vi "CreateShift.vi"(7 "Shifter Name":string, 8 "error in (no error)":errorcluster, 9 "Duration Hours":u8, 10 "Start Hour":u8, 11 "Date":string) -> (0 "error out":errorcluster, 3 "Shift":refnum<class "Shift.lvclass">)   [LabVIEW 2013, in "Shift Schedule.lvclass"]
uses:
  Shift Schedule.lvclass
  Shift.lvclass
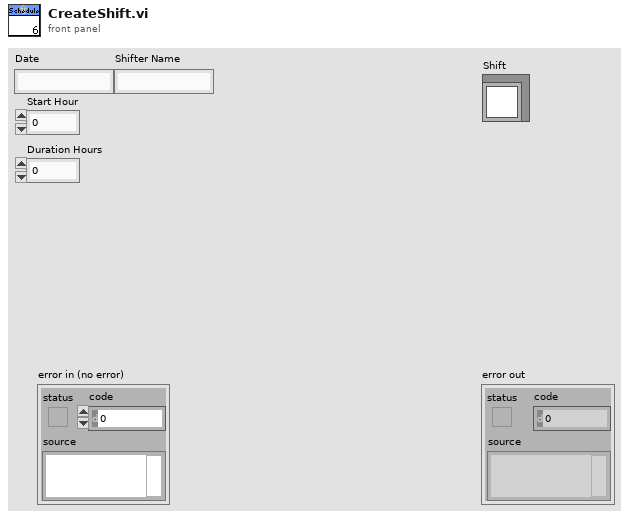
[diagram p1: front panel]
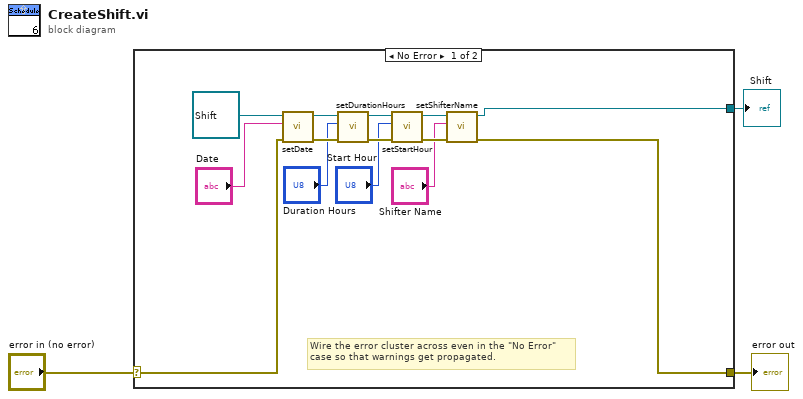
[diagram p0: block diagram]
diagram:
  n1 = case shown="No Error" "error in (no error)" {
    selector: "error in (no error)" -> [w13 w18]
    tunnel: [w7 w18] -> w2
    tunnel: [w8 _] -> w1
    frame No Error {
      # "Wire the error cluster across even in the \"No Error\"\ncase so that warnings get propagated."
      n2 = call-dynamic "setDate.vi"("error in (no error)"=w13, "Date"="Date", "Shift in"=refnum<class "Shift.lvclass"> refnum ("Shift.lvclass")) -> ("error out"=w14:errorcluster, "Shift out"=w15:refnum<class "Shift.lvclass">)  [unwired: 7 in]
      n3 = call-dynamic "setDurationHours.vi"("error in (no error)"=w14, "Duration Hours"="Duration Hours", "Shift in"=w15) -> ("error out"=w12:errorcluster, "Shift out"=w10:refnum<class "Shift.lvclass">)  [unwired: 7 in]
      n4 = call-dynamic "setStartHour.vi"("error in (no error)"=w12, "Start Hour"="Start Hour", "Shift in"=w10) -> ("error out"=w11:errorcluster, "Shift out"=w9:refnum<class "Shift.lvclass">)  [unwired: 7 in]
      n5 = call-dynamic "setShifterName.vi"("error in (no error)"=w11, "Shifter Name"="Shifter Name", "Shift in"=w9) -> ("error out"=w7:errorcluster, "Shift out"=w8:refnum<class "Shift.lvclass">)  [unwired: 7 in]
    }
    frame Error {
    }
  }
  "error out" <- w2
  "Shift" <- w1
